vi "Feedbacks gradients.vi"(1 "Wavenet, Z":dbl[][](array[numeric]) format="%.3f", 2 "Identification errors, e":dbl[][](array[numeric]) format="%.3f", 3 "Total control, U":dbl=1.0 min=1.0 max=10.0 step=1.0 format="%.3f") -> (0 "Feedbacks, C":dbl[][](array[numeric]) format="%.3f")   [LabVIEW 2022 SP3]
uses:
  <vilib>/Analysis/baseanly.llb/Real A x B.vi
  <vilib>/Analysis/NI_AALBase.lvlib
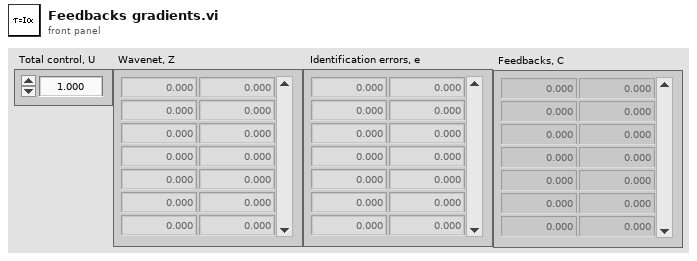
[diagram p1: front panel]
types:
  T1 = typedef "NI_Matrix.lvlib/RealMatrix.ctl" = dbl[][]
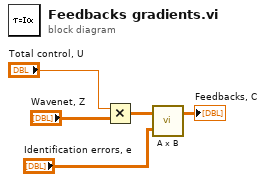
[diagram p0: block diagram]
diagram:
  n1 = Multiply(x="Total control, U", y="Wavenet, Z") -> (x*y=w4:dbl[][])
  n2 = call-poly <vilib>:"A x B.vi"("B"="Identification errors, e", "A"=w4) -> ("A x B"=→"Feedbacks, C":T1)  [unwired: 1 out]
